vi "cDAQ_M.vi"(8 "error in":errorcluster) -> (0 "error out":errorcluster, 3 "task out":refnum<k21>)   [LabVIEW 2022 SP3]
uses:
  <vilib>/DAQmx/create/channels.llb/DAQmx Create Channel (AI-Voltage-Basic).vi
  <vilib>/DAQmx/create/channels.llb/DAQmx Create Channel (AI-Current-Basic).vi
  <vilib>/DAQmx/configure/timing.llb/DAQmx Timing (Sample Clock).vi
  <resource>/objmgr/daqmx.rc
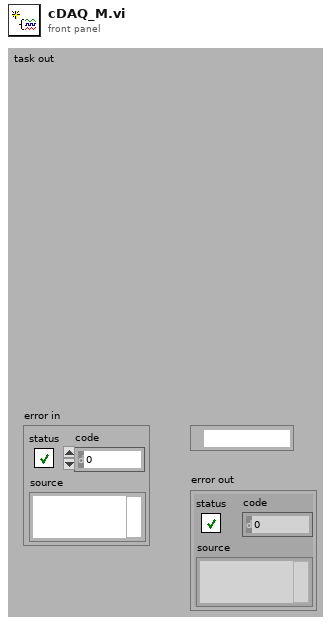
[diagram p1: front panel]
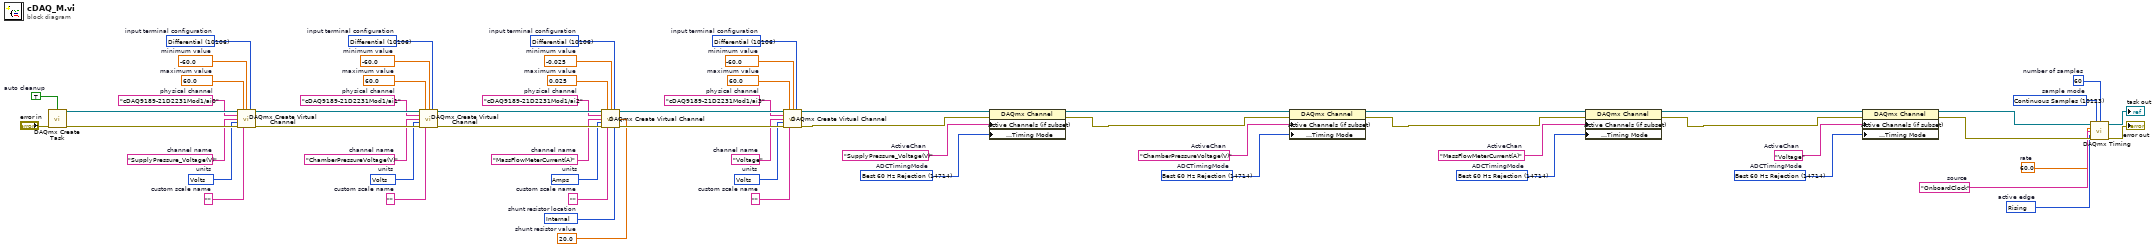
[diagram p0: block diagram]
diagram:
  w1 = 10123 items=["Finite Samples"=10178, "Continuous Samples"=10123, "Hardware Timed Single Point"=12522]  # sample mode
  w2 = 60.0  # rate
  w3 = 10280 items=["Rising"=10280, "Falling"=10171]  # active edge
  w4 = "OnboardClock"  # source
  w5 = 60  # number of samples
  w10 = 14714 items=["High Resolution"=10195, "High Speed"=14712, "Best 50 Hz Rejection"=14713, "Best 60 Hz Rejection"=14714]  # ADCTimingMode
  w12 = "Voltage"  # ActiveChan
  w14 = 14714 items=["High Resolution"=10195, "High Speed"=14712, "Best 50 Hz Rejection"=14713, "Best 60 Hz Rejection"=14714]  # ADCTimingMode
  w16 = "MassFlowMeterCurrent(A)"  # ActiveChan
  w18 = 14714 items=["High Resolution"=10195, "High Speed"=14712, "Best 50 Hz Rejection"=14713, "Best 60 Hz Rejection"=14714]  # ADCTimingMode
  w20 = "ChamberPressureVoltage(V)"  # ActiveChan
  w22 = 14714 items=["High Resolution"=10195, "High Speed"=14712, "Best 50 Hz Rejection"=14713, "Best 60 Hz Rejection"=14714]  # ADCTimingMode
  w24 = "SupplyPressure_Voltage(V)"  # ActiveChan
  w25 = 10106 items=["default"=-1, "RSE"=10083, "NRSE"=10078, "Differential"=10106, "Pseudodifferential"=12529]  # input terminal configuration
  w26 = 10348 items=["Volts"=10348, "From Custom Scale"=10065]  # units
  w27 = "Voltage"  # channel name
  w29 = ""  # custom scale name
  w30 = -60.0  # minimum value
  w31 = 60.0  # maximum value
  w32 = "cDAQ9189-21D2231Mod1/ai3"  # physical channel
  w34 = 10106 items=["default"=-1, "RSE"=10083, "NRSE"=10078, "Differential"=10106, "Pseudodifferential"=12529]  # input terminal configuration
  w35 = 10342 items=["Amps"=10342, "From Custom Scale"=10065]  # units
  w36 = 20.0  # shunt resistor value
  w37 = 10200 items=["Internal"=10200, "External"=10167]  # shunt resistor location
  w38 = "MassFlowMeterCurrent(A)"  # channel name
  w40 = ""  # custom scale name
  w41 = -0.025  # minimum value
  w42 = 0.025  # maximum value
  w43 = "cDAQ9189-21D2231Mod1/ai2"  # physical channel
  w45 = 10106 items=["default"=-1, "RSE"=10083, "NRSE"=10078, "Differential"=10106, "Pseudodifferential"=12529]  # input terminal configuration
  w46 = 10348 items=["Volts"=10348, "From Custom Scale"=10065]  # units
  w47 = "ChamberPressureVoltage(V)"  # channel name
  w49 = ""  # custom scale name
  w50 = -60.0  # minimum value
  w51 = 60.0  # maximum value
  w52 = "cDAQ9189-21D2231Mod1/ai1"  # physical channel
  w54 = 10106 items=["default"=-1, "RSE"=10083, "NRSE"=10078, "Differential"=10106, "Pseudodifferential"=12529]  # input terminal configuration
  w55 = 10348 items=["Volts"=10348, "From Custom Scale"=10065]  # units
  w56 = "SupplyPressure_Voltage(V)"  # channel name
  w58 = ""  # custom scale name
  w59 = -60.0  # minimum value
  w60 = 60.0  # maximum value
  w61 = "cDAQ9189-21D2231Mod1/ai0"  # physical channel
  w63 = TRUE  # auto cleanup
  n1 = call <vilib>:"DAQmx Create Task.vi"("auto cleanup"=w63, "error in"="error in") -> ("task out"=w62:refnum<k21>, "error out"=w64:errorcluster)  [unwired: 12 in]
  n2 = call-poly <vilib>:"DAQmx Create Virtual Channel.vi"("task in"=w62, "maximum value"=w60, "minimum value"=w59, "input terminal configuration"=w54, "physical channels"=w61, "name to assign"=w56, "units"=w55, "error in"=w64, "custom scale name"=w58) -> ("task out"=w53:refnum<k21>, "error out"=w57:errorcluster)  [unwired: 5 in]
  n3 = call-poly <vilib>:"DAQmx Create Virtual Channel.vi"("task in"=w53, "maximum value"=w51, "minimum value"=w50, "input terminal configuration"=w45, "physical channels"=w52, "name to assign"=w47, "units"=w46, "error in"=w57, "custom scale name"=w49) -> ("task out"=w44:refnum<k21>, "error out"=w48:errorcluster)  [unwired: 5 in]
  n4 = call-poly <vilib>:"DAQmx Create Virtual Channel.vi"("task in"=w44, "maximum value"=w42, "minimum value"=w41, "input terminal configuration"=w34, "physical channels"=w43, "name to assign"=w38, "external shunt resistor value"=w36, "units"=w35, "error in"=w48, "custom scale name"=w40, "shunt resistor location"=w37) -> ("task out"=w33:refnum<k21>, "error out"=w39:errorcluster)  [unwired: 3 in]
  n5 = call-poly <vilib>:"DAQmx Create Virtual Channel.vi"("task in"=w33, "maximum value"=w31, "minimum value"=w30, "input terminal configuration"=w25, "physical channels"=w32, "name to assign"=w27, "units"=w26, "error in"=w39, "custom scale name"=w29) -> ("task out"=w21:refnum<k21>, "error out"=w28:errorcluster)  [unwired: 5 in]
  n6 = property class="DAQmx Channel"(reference=w21, error in=w28, "Active Channels (if subset)"=w24, "Analog Input:General Properties:Digitizer/ADC:Timing Mode"=w22) -> (reference out=w17:refnum<k21>, error out=w23:errorcluster)
  n7 = property class="DAQmx Channel"(reference=w17, error in=w23, "Active Channels (if subset)"=w20, "Analog Input:General Properties:Digitizer/ADC:Timing Mode"=w18) -> (reference out=w13:refnum<k21>, error out=w19:errorcluster)
  n8 = property class="DAQmx Channel"(reference=w13, error in=w19, "Active Channels (if subset)"=w16, "Analog Input:General Properties:Digitizer/ADC:Timing Mode"=w14) -> (reference out=w9:refnum<k21>, error out=w15:errorcluster)
  n9 = property class="DAQmx Channel"(reference=w9, error in=w15, "Active Channels (if subset)"=w12, "Analog Input:General Properties:Digitizer/ADC:Timing Mode"=w10) -> (reference out=w6:refnum<k21>, error out=w11:errorcluster)
  n10 = call-poly <vilib>:"DAQmx Timing.vi"("task/channels in"=w6, "sample mode"=w1, "samples per channel"=w5, "rate"=w2, "source"=w4, "active edge"=w3, "error in"=w11) -> ("task out"=→"task out":refnum<k21>, "error out"=→"error out":errorcluster)  [unwired: 7 in]
